vi "Shared Set Object Pointer.vi"(10 "Object Pointer":i64, 11 "Tree in":refnum<class "Tree.lvclass">) -> (3 "Tree out":refnum<class "Tree.lvclass">)   [LabVIEW 2012, in "MDSplus.lvlib" / "Tree.lvclass"]
uses:
  <vilib>/MDSplus/Classes/Tree_Class/Tree.lvclass
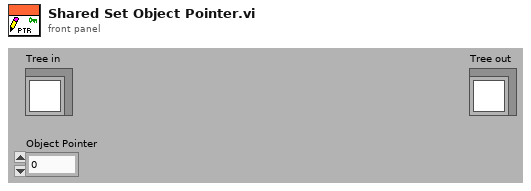
[diagram p1: front panel]
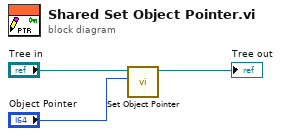
[diagram p0: block diagram]
diagram:
  n1 = call-dynamic "Set Object Pointer.vi"("Object Pointer"="Object Pointer", "Tree in"="Tree in") -> ("Tree out"=→"Tree out":refnum<class "Tree.lvclass">)  [unwired: 9 in]
